vi "CheckHardware.vi"(8 "error in":errorcluster, 11 "CpuFeatures":T1 items=["CPU_MMX            "=1, "CPU_SSE            "=2, "CPU_SSE2           "=3, "CPU_SSE3           "=4, "CPU_SSSE3          "=5, "CPU_SSE4_1         "=6, "CPU_SSE4_2         "=7, "CPU_POPCNT         "=8, "CPU_FP16           "=9, "CPU_AVX            "=10, "CPU_AVX2           "=11, "CPU_FMA3           "=12, "CPU_AVX_512F       "=13, "CPU_AVX_512BW      "=14, "CPU_AVX_512CD      "=15, "CPU_AVX_512DQ      "=16, "CPU_AVX_512ER      "=17, "CPU_AVX_512IFMA    "=18, "CPU_AVX_512PF      "=19, "CPU_AVX_512VBMI    "=20, "CPU_AVX_512VL      "=21, "CPU_AVX_512VBMI2   "=22, "CPU_AVX_512VNNI    "=23, "CPU_AVX_512BITALG  "=24, "CPU_AVX_512VPOPCNTDQ"=25, "CPU_AVX_5124VNNIW  "=26, "CPU_AVX_5124FMAPS  "=27, "CPU_NEON           "=100, "CPU_NEON_DOTPROD   "=101, "CPU_NEON_FP16      "=102, "CPU_NEON_BF16      "=103, "CPU_MSA            "=150, "CPU_RISCVV         "=170, "CPU_VSX            "=200, "CPU_VSX3           "=201, "CPU_RVV            "=210, "CPU_LSX            "=230, "CPU_LASX           "=231, "CPU_AVX512_SKX     "=256, "CPU_AVX512_COMMON  "=257, "CPU_AVX512_KNL     "=258, "CPU_AVX512_KNM     "=259, "CPU_AVX512_CNL     "=260, "CPU_AVX512_CLX     "=261, "CPU_AVX512_ICL     "=262, "CPU_MAX_FEATURE    "=512]) -> (0 "error out":errorcluster, 3 "isSupported":bool)   [LabVIEW 2020, in "OpenLvVision_OpenCv.lvlib"]
doc: "The function returns true if the host hardware supports the specified feature. When user calls setUseOptimized(false), the subsequent calls to checkHardwareSupport() will return false until setUseOptimized(true) is called. This way user can dynamically switch on and off the optimized code in OpenCV."
uses:
  OpenLvVision_OpenCv.lvlib
  TypeDef/CpuFeatures.ctl
  Dlls/OlvOpenCvWrapper.dll
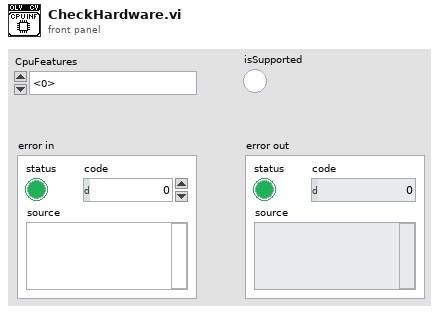
[diagram p1: front panel]
types:
  T1 = typedef "OpenLvVision_OpenCv.lvlib/CpuFeatures.ctl" = i32
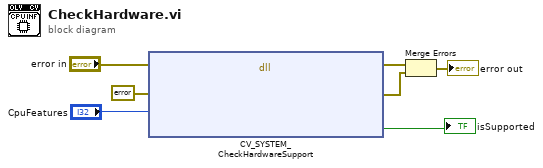
[diagram p0: block diagram]
diagram:
  n1 = dll-call lib="C:/Users/lukas/Downloads/OpenLvVision_OpenCv/SourceCode/LabView/OpenLvVision_OpenCv/Dlls/OlvOpenCvWrapper.dll" fn="CV_SYSTEM_CheckHardwareSupport"(error in="error in", "Error"=errorcluster {"status"=FALSE, "code"=0, "source"=""} ("error in"), "featureID"="CpuFeatures") -> (error out=w5:errorcluster, "Error"=w3:errorcluster, "isSupported"=→"isSupported":bool)  [unwired: 5 in, 1 out]
  n2 = Merge Errors(w5, w3) -> (→"error out":errorcluster)
